vi "ex_readTdmChannelInfo.vi"(3 "error in (no error)":errorcluster, 4 "read info in":T4) -> (0 "error out":errorcluster, 1 "read info out":T4, 2 "comment":string)   [LabVIEW 2017]
uses:
  <vilib>/Platform/express/TDMExpress.llb/ex_readInfoTDM.ctl
  <vilib>/Platform/express/TDMExpress.llb/ex_readChannelInfo.ctl
  <vilib>/express/express shared/ExFile.llb/ex_TdmData.ctl
  <vilib>/express/express shared/ExFile.llb/ex_TdmProperty.ctl
  <vilib>/express/express shared/ex_EditUserDefinedProperties/usiDataType.ctl
  <vilib>/Platform/storage/lvStorage.llb/_wf_attributes.ctl
  <vilib>/Platform/storage/Storage.llb/__loadPropString.vi
  <vilib>/Platform/storage/Storage.llb/__loadPropRefList.vi
  <vilib>/Platform/storage/Storage.llb/__loadPropFloat64.vi
  <vilib>/Platform/storage/Storage.llb/__loadPropTime.vi
panel:
  out "Array":T1(array[cluster])
  in  "channel info":T2={"data chn ref"=refnum, "time chn ref"=refnum, "isRelativeTime ?"=FALSE, "channel length"=0, "dT"=0.0, "waveform stub"={"t0"=timestamp(0 s since 1904-01-01), "dt"=0.0, "Y"=[]}, "datatype"="", "timestamp"=timestamp(0 s since 1904-01-01)}
  in  "All Express Wave Attributes Plus PLUS":T3={"Start Timestamp"=timestamp(3198762007.7559996 s since 1904-01-01), "Timestamp"=timestamp(3198762007.8559995 s since 1904-01-01), "Relative Time?"=TRUE, "X Dimension"="f", "Signal Name"="Sawtooth with Uniform Noise (Power Spectrum)", "Y Units"="", "X0"=timestamp(0 s since 1904-01-01), "dX"=10.0, "nPoints"=50, "refnum"=refnum, "datatype"=""} {"dX" format="%.2f"; "X0" format="%<%X\n%x>T"; "Timestamp" format="%<%X\n%x>T"; "Start Timestamp" format="%<%X\n%x>T"}
  in  "Empty waveform":waveform(dbl)
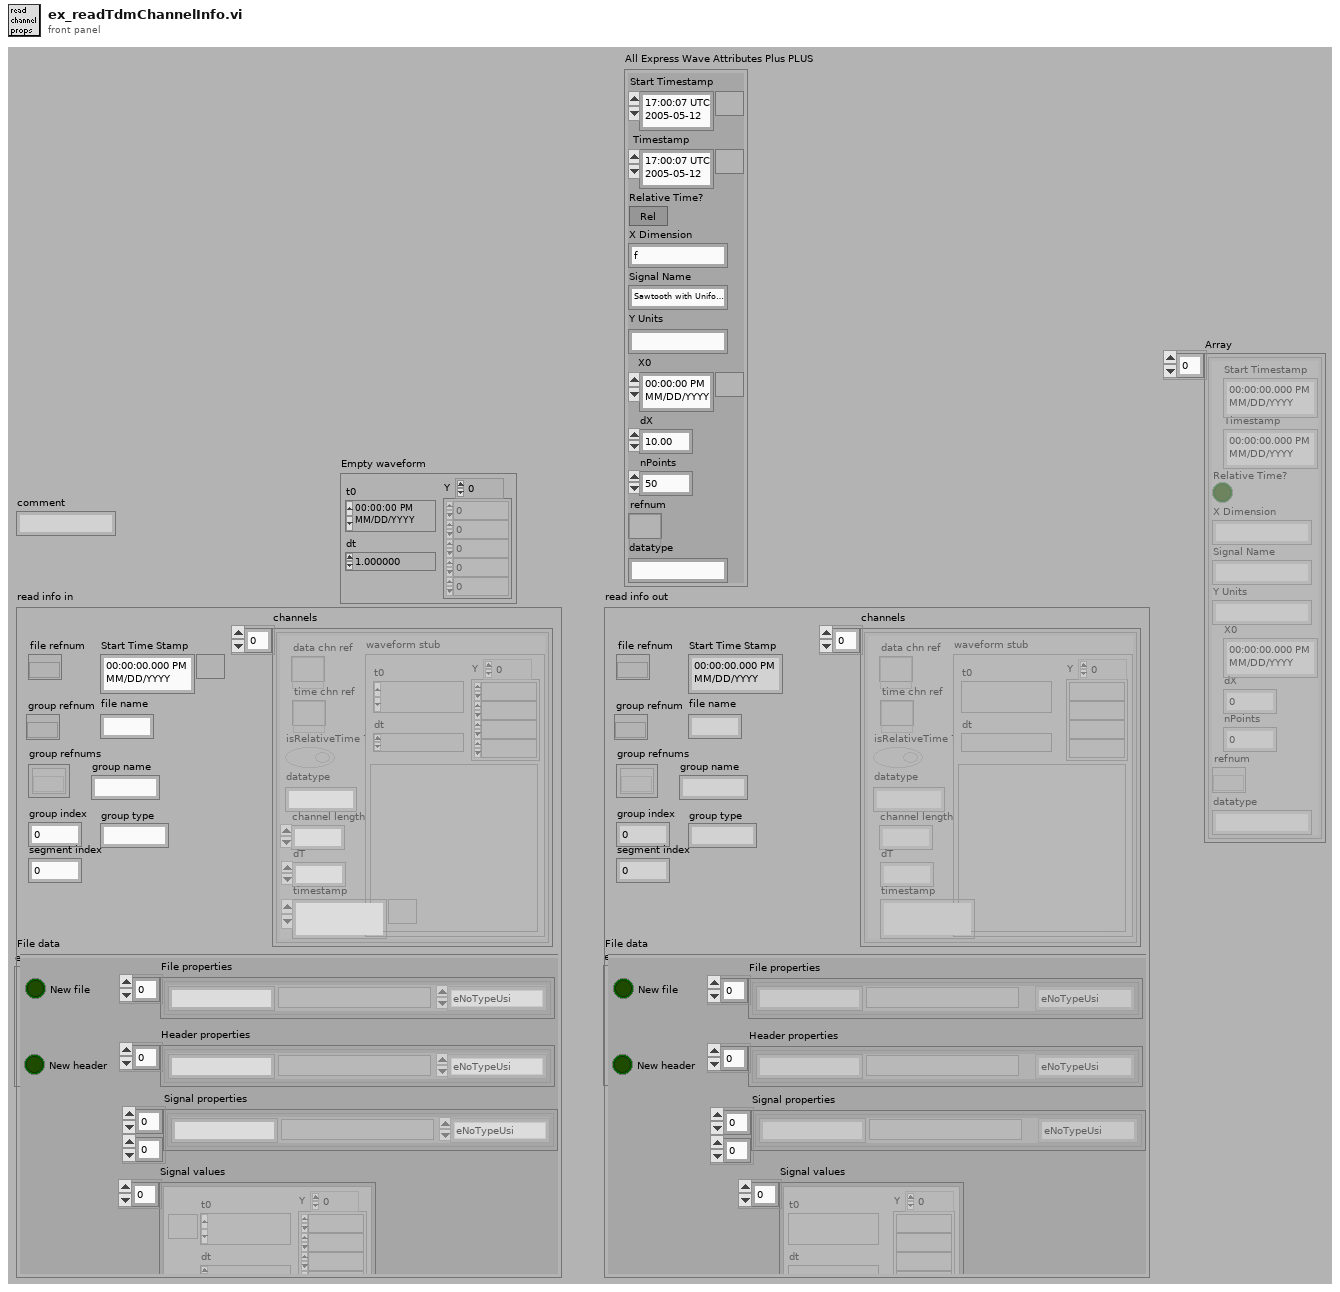
[diagram p1: front panel]
types:
  T1 = cluster{"Start Timestamp":timestamp, "Timestamp":timestamp, "Relative Time?":bool, "X Dimension":string, "Signal Name":string, "Y Units":string, "X0":timestamp, "dX":dbl, "nPoints":i32, "refnum":refnum<k20>, "datatype":string}[]
  T2 = typedef "ex_readChannelInfo.ctl" = cluster{"data chn ref":refnum<k20>, "time chn ref":refnum<k20>, "isRelativeTime ?":bool, "channel length":u32, "dT":dbl, "waveform stub":waveform(dbl), "datatype":string, "timestamp":timestamp}
  T3 = cluster{"Start Timestamp":timestamp, "Timestamp":timestamp, "Relative Time?":bool, "X Dimension":string, "Signal Name":string, "Y Units":string, "X0":timestamp, "dX":dbl, "nPoints":i32, "refnum":refnum<k20>, "datatype":string}
  T4 = typedef "ex_readInfoTDM.ctl" = cluster{"file refnum":refnum<k20>, "group refnum":refnum<k20>, "group name":string, "group type":string, "Start Time Stamp":timestamp, "group index":u32, "group refnums":refnum<k20>[], "file name":string, "segment index":u32, "channels":T2[], "File data":T5}
  T5 = typedef "ex_TdmData.ctl" = cluster{"New file":bool, "New header":bool, "File properties":T6[], "Header properties":T6[], "Signal properties":T6[][], "Signal values":waveform(dbl)[]}
  T6 = typedef "ex_TdmProperty.ctl" = cluster{"Name":string, "Type":T7, "Value":variant}
  T7 = typedef "usiDataType.ctl" = enum16{"eNoTypeUsi", "eInt8Usi", "eInt16Usi", "eInt32Usi", "eInt64Usi", "eUInt8Usi", "eUInt16Usi", "eUInt32Usi", "eUInt64Usi", "eFloat32Usi", "eFloat64Usi", "- 0", "- 1", "- 2", "- 3", "- 4", "- 5", "- 6", "- 7", "- 8", "- 9", "eString8Usi", "eString16Usi", "eStringUsi", "eEnumUsi", "- 10", "- 11", "- 12", "- 13", "- 14", "eTimeUsi", "- 15", "- 16", "- 17", "- 18", "- 19", "- 20", "- 21", "- 22", "- 23", "eInstanceUsi", "eStoreUsi"}
  T8 = typedef "_wf_attributes.ctl" = enum16{"t0", "dt", "X_Name", "X_Unit", "x0", "abs/rel", "nPoints", "file_timestamp", "xcolumns"}
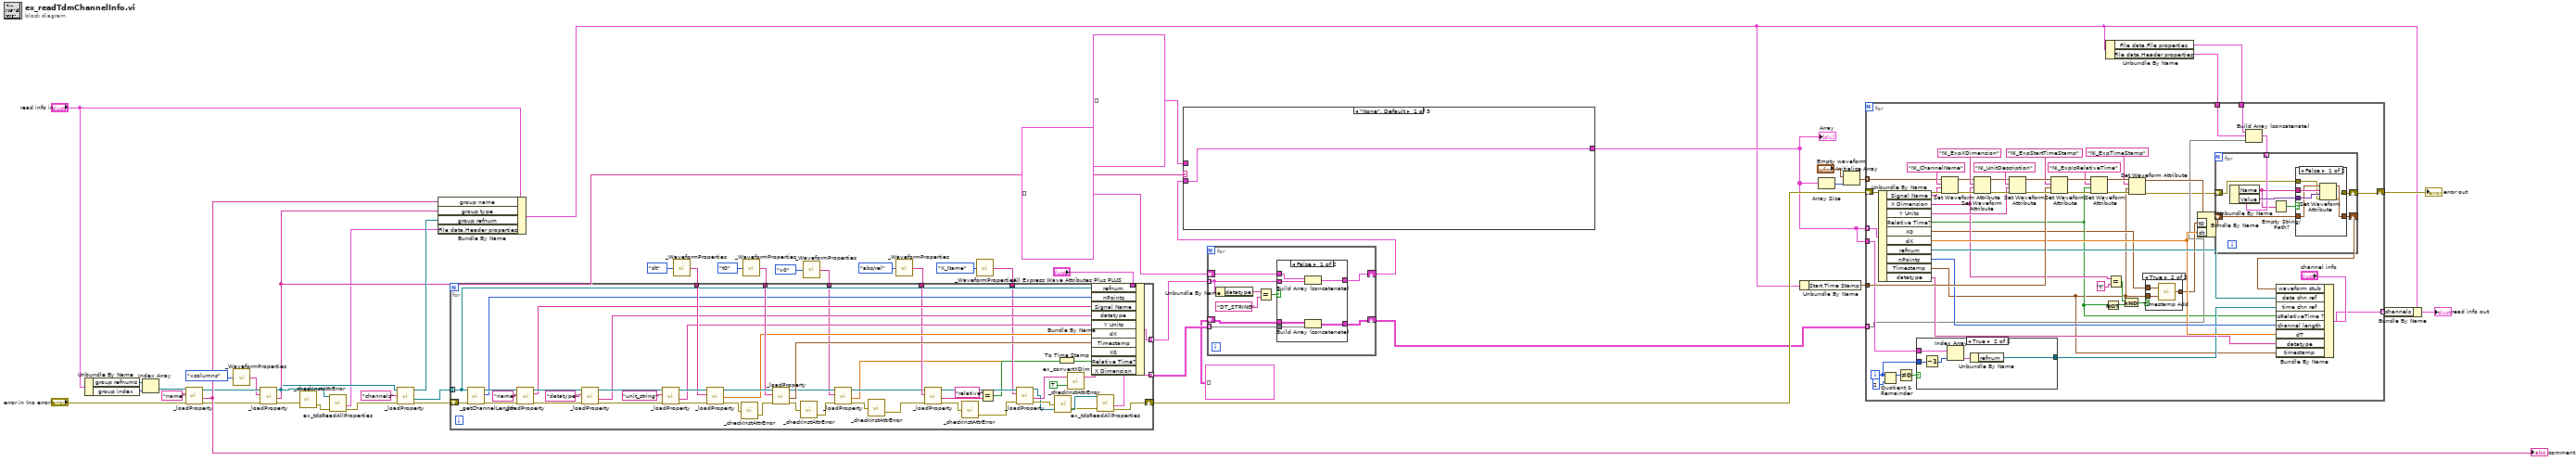
[diagram p0: block diagram]
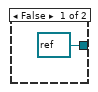
[diagram p5: hidden frame]
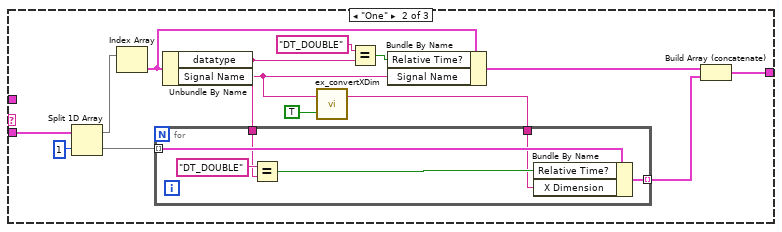
[diagram p6: hidden frame]
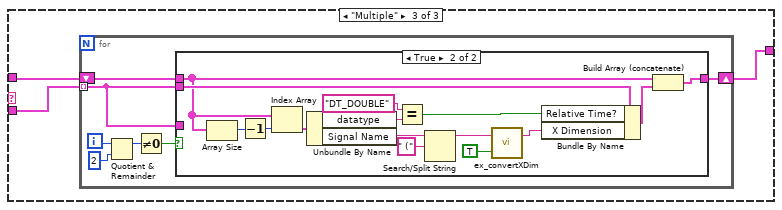
[diagram p7: hidden frame]
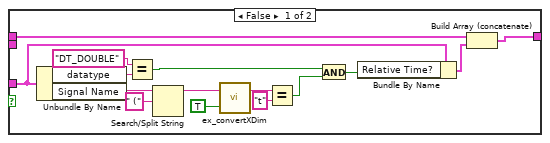
[diagram p8: hidden frame]
diagram:
  n1 = Unbundle By Name("read info in") -> ("group refnums"=w41:refnum<k20>[], "group index"=w50:u32)
  n2 = Index Array(array=w41, index=w50) -> (element=w42:refnum<k20>)
  n3 = call-poly <vilib>:"_loadProperty.vi"("error in (no error)"="error in (no error)", "Property name"="name", "storage refnum"=w42) -> ("error out"=w45:errorcluster, "Value"=w51:string, "dup storage refnum"=w46:refnum<k20>)  [unwired: 6 out]
  "comment" <- w51
  n4 = call <vilib>:"_WaveformProperties.vi"("Property"=_wf_attributes."xcolumns") -> ("Name"=w43:string)
  n5 = call-poly <vilib>:"_loadProperty.vi"("error in (no error)"=w45, "Property name"=w43, "storage refnum"=w46) -> ("error out"=w18:errorcluster, "Value"=w36:string, "dup storage refnum"=w14:refnum<k20>)  [unwired: 6 out]
  n6 = call <vilib>:"_checkInstAttrError.vi"("error in (no error)"=w18) -> ("error out"=w13:errorcluster)  [unwired: 1 out]
  n7 = call <vilib>:"ex_tdsReadAllProperties.vi"("error in (no error)"=w13, "Data Object in"=w14) -> ("error out"=w12:errorcluster, "Properties Out"=w11:T6[])  [unwired: 4 out]
  n8 = call-poly <vilib>:"_loadProperty.vi"("error in (no error)"=w12, "Property name"="channels", "storage refnum"=w14) -> ("error out"=w39:errorcluster, "Value"=w40:refnum<k20>[], "dup storage refnum"=w38:refnum<k20>)  [unwired: 6 out]
  n9 = Bundle By Name(cluster="read info in", "group name"=w51, "group type"=w36, "group refnum"=w38, "File data.Header properties"=w11) -> (w9:T4)
  n10 = call <vilib>:"_WaveformProperties.vi"("Property"=_wf_attributes."dt") -> ("Name"=w27:string)
  n11 = call <vilib>:"_WaveformProperties.vi"("Property"=_wf_attributes."t0") -> ("Name"=w25:string)
  n12 = call <vilib>:"_WaveformProperties.vi"("Property"=_wf_attributes."x0") -> ("Name"=w15:string)
  n13 = call <vilib>:"_WaveformProperties.vi"("Property"=_wf_attributes."abs/rel") -> ("Name"=w22:string)
  n14 = call <vilib>:"_WaveformProperties.vi"("Property"=_wf_attributes."X_Name") -> ("Name"=w19:string)
  n15 = for {
    shift-right: [w53] -> w32
    shift-left: w39 -> [w102]
    tunnel: w40 -> [w76] mode=indexing
    tunnel: w27 -> [w91]
    tunnel: w25 -> [w89]
    tunnel: "All Express Wave Attributes Plus PLUS" -> [w87]
    tunnel: w22 -> [w80]
    tunnel: [w77] -> w5 mode=indexing
    tunnel: w19 -> [w74]
    tunnel: w15 -> [w59]
    tunnel: [w52] -> w3 mode=indexing
    n16 = call <vilib>:"_getChannelLength.vi"("error in (no error)"=w102, "channel refnum in"=w76) -> ("error out"=w99:errorcluster, "channel length"=w86:i32, "channel refnum out"=w98:refnum<k20>)  [unwired: 3 out]
    n17 = call-poly <vilib>:"_loadProperty.vi"("error in (no error)"=w99, "Property name"="name", "storage refnum"=w98) -> ("error out"=w97:errorcluster, "Value"=w85:string, "dup storage refnum"=w96:refnum<k20>)  [unwired: 1 in, 5 out]
    n18 = call-poly <vilib>:"_loadProperty.vi"("error in (no error)"=w97, "Property name"="datatype", "storage refnum"=w96) -> ("error out"=w94:errorcluster, "Value"=w84:string, "dup storage refnum"=w93:refnum<k20>)  [unwired: 1 in, 5 out]
    n19 = call-poly <vilib>:"_loadProperty.vi"("error in (no error)"=w94, "Property name"="unit_string", "storage refnum"=w93) -> ("error out"=w88:errorcluster, "Value"=w83:string, "dup storage refnum"=w92:refnum<k20>)  [unwired: 1 in, 5 out]
    n20 = call-poly <vilib>:"_loadProperty.vi"("error in (no error)"=w88, "Property name"=w91, "storage refnum"=w92) -> ("error out"=w70:errorcluster, "Value"=w82:dbl, "dup storage refnum"=w90:refnum<k20>)  [unwired: 6 out]
    n21 = call <vilib>:"_checkInstAttrError.vi"("error in (no error)"=w70) -> ("error out"=w69:errorcluster)  [unwired: 1 out]
    n22 = call-poly <vilib>:"_loadProperty.vi"("error in (no error)"=w69, "Property name"=w89, "storage refnum"=w90) -> ("error out"=w68:errorcluster, "Value"=w81:timestamp, "dup storage refnum"=w61:refnum<k20>)  [unwired: 6 out]
    n23 = call <vilib>:"_checkInstAttrError.vi"("error in (no error)"=w68) -> ("error out"=w63:errorcluster)  [unwired: 1 out]
    n24 = call-poly <vilib>:"_loadProperty.vi"("error in (no error)"=w63, "Property name"=w59, "storage refnum"=w61) -> ("error out"=w64:errorcluster, "Value"=w56:dbl, "dup storage refnum"=w60:refnum<k20>)  [unwired: 6 out]
    n25 = call <vilib>:"_checkInstAttrError.vi"("error in (no error)"=w64) -> ("error out"=w62:errorcluster)  [unwired: 1 out]
    n26 = call-poly <vilib>:"_loadProperty.vi"("error in (no error)"=w62, "Property name"=w80, "storage refnum"=w60) -> ("error out"=w67:errorcluster, "Value"=w79:string, "dup storage refnum"=w75:refnum<k20>)  [unwired: 6 out]
    n27 = call <vilib>:"_checkInstAttrError.vi"("error in (no error)"=w67) -> ("error out"=w66:errorcluster)  [unwired: 1 out]
    n28 = Equal?(x="relative", y=w79) -> (x = y?=w58:bool)
    n29 = call-poly <vilib>:"_loadProperty.vi"("error in (no error)"=w66, "Property name"=w74, "storage refnum"=w75) -> ("error out"=w65:errorcluster, "Value"=w72:string, "dup storage refnum"=w55:refnum<k20>)  [unwired: 6 out]
    n30 = call <vilib>:"_checkInstAttrError.vi"("error in (no error)"=w65) -> ("error out"=w54:errorcluster)  [unwired: 1 out]
    n31 = To Time Stamp(1:w56) -> (0:w57:timestamp)
    n32 = call <vilib>:"ex_convertXDim.vi"("mode (F:Code to String)"=TRUE, "x_dimension in"=w72) -> ("x_dimension out"=w71:string)  [unwired: 1 out]
    n33 = Bundle By Name(cluster=w87, "refnum"=w76, "nPoints"=w86, "Signal Name"=w85, "datatype"=w84, "Y Units"=w83, "dX"=w82, "Timestamp"=w81, "X0"=w57, "Relative Time?"=w58, "X Dimension"=w71) -> (w77:T3)
    n34 = call <vilib>:"ex_tdsReadAllProperties.vi"("error in (no error)"=w54, "Data Object in"=w55) -> ("error out"=w53:errorcluster, "Properties Out"=w52:T6[])  [unwired: 4 out]
  }
  n35 = for {
    tunnel: w5 -> [w108] mode=indexing
    shift-right: [w107] -> w4
    shift-left: T1 [] ("Array 2") -> [w106]
    tunnel: w3 -> [w105] mode=indexing
    shift-right: [w104] -> w1
    shift-left: T6[][] [] ("Properties Out") -> [w103]
    n36 = Unbundle By Name(w108) -> ("datatype"=w111:string)
    n37 = Equal?(x=w111, y="DT_STRING") -> (x = y?=w109:bool)
    n38 = case shown="False" w109 {
      tunnel: w108 -> [w117 _]
      tunnel: [w116 w119] -> w107
      tunnel: w106 -> [w115 w119]
      tunnel: w105 -> [w114 _]
      tunnel: [w113 w118] -> w104
      tunnel: w103 -> [w112 w118]
      frame False {
        n39 = Build Array (concatenate)(w115, w117) -> (w116:T1)
        n40 = Build Array (concatenate)(w112, w114) -> (w113:T6[][])
      }
      frame True {
      }
    }
  }
  n41 = case shown="\"None\", Default" w36 {
    tunnel: w4 -> [w120 w132 w142]
    tunnel: [w120 w123 w141] -> w10
    tunnel: T1 [] -> [_ _ w143]
    frame "None", Default {
    }
    frame "One" {
      n42 = Split 1D Array(array=w132, index=1) -> (first subarray=w131:T1, second subarray=w129:T1)
      n43 = Index Array(array=w131) -> (element=w130:T3)  [unwired: 1 in]
      n44 = Unbundle By Name(w130) -> ("datatype"=w127:string, "Signal Name"=w121:string)
      n45 = call <vilib>:"ex_convertXDim.vi"("mode (F:Code to String)"=TRUE, "x_dimension in"=w121) -> ("x_dimension out"=w125:string)  [unwired: 1 out]
      n46 = for {
        tunnel: w129 -> [w140] mode=indexing
        tunnel: [w138] -> w124 mode=indexing
        tunnel: w127 -> [w136]
        tunnel: w125 -> [w135]
        n47 = Equal?(x="DT_DOUBLE", y=w136) -> (x = y?=w139:bool)
        n48 = Bundle By Name(cluster=w140, "Relative Time?"=w139, "X Dimension"=w135) -> (w138:T3)
      }
      n49 = Equal?(x="DT_DOUBLE", y=w127) -> (x = y?=w126:bool)
      n50 = Bundle By Name(cluster=w130, "Relative Time?"=w126, "Signal Name"=w121) -> (w122:T3)
      n51 = Build Array (concatenate)(w122, w124) -> (w123:T1)
    }
    frame "Multiple" {
      n52 = for {
        shift-right: [w147] -> w141
        shift-left: w143 -> [w148]
        tunnel: w142 -> [w145] mode=indexing
        i -> [w144]
        n53 = Quotient & Remainder(x=w144, y=2) -> (x-y*floor(x/y)=w146:i32)  [unwired: 1 out]
        n54 = Not Equal To 0?(x=w146) -> (x != 0?=w149:bool)
        n55 = case shown="True" w149 {
          tunnel: w148 -> [w157 w171]
          tunnel: [w156 w180] -> w147
          tunnel: w145 -> [_ w177]
          tunnel: w145 -> [w158 _]
          frame False {
            n56 = Unbundle By Name(w158) -> ("datatype"=w164:string, "Signal Name"=w160:string)
            n57 = Equal?(x="DT_DOUBLE", y=w164) -> (x = y?=w155:bool)
            n58 = Search/Split String(string=w160, search string/char (-)=" (") -> (substring before match=w163:string)  [unwired: 3 out]
            n59 = call <vilib>:"ex_convertXDim.vi"("mode (F:Code to String)"=TRUE, "x_dimension in"=w163) -> ("x_dimension out"=w153:string)  [unwired: 1 out]
            n60 = Equal?(x=w153, y="t") -> (x = y?=w152:bool)
            n61 = And(x=w155, y=w152) -> (x .and. y?=w154:bool)
            n62 = Bundle By Name(cluster=w158, "Relative Time?"=w154) -> (w159:T3)
            n63 = Build Array (concatenate)(w157, w159) -> (w156:T1)
          }
          frame True {
            n64 = Array Size(array=w171) -> (size(s)=w172:i32)
            n65 = Decrement(x=w172) -> (x-1=w175:i32)
            n66 = Index Array(array=w171, index=w175) -> (element=w174:T3)
            n67 = Unbundle By Name(w174) -> ("datatype"=w173:string, "Signal Name"=w167:string)
            n68 = Equal?(x="DT_DOUBLE", y=w173) -> (x = y?=w178:bool)
            n69 = Search/Split String(string=w167, search string/char (-)=" (") -> (substring before match=w170:string)  [unwired: 3 out]
            n70 = call <vilib>:"ex_convertXDim.vi"("mode (F:Code to String)"=TRUE, "x_dimension in"=w170) -> ("x_dimension out"=w166:string)  [unwired: 1 out]
            n71 = Bundle By Name(cluster=w177, "Relative Time?"=w178, "X Dimension"=w166) -> (w176:T3)
            n72 = Build Array (concatenate)(w171, w176) -> (w180:T1)
          }
        }
      }
    }
  }
  "Array" <- w10
  n73 = Unbundle By Name(w9) -> ("Start Time Stamp"=w30:timestamp)
  n74 = Array Size(array=w10) -> (size(s)=w35:i32)
  n75 = Initialize Array("Empty waveform", w35) -> (w33:waveform(dbl)[])
  n76 = Unbundle By Name(w9) -> ("File data.File properties"=w8:T6[], "File data.Header properties"=w7:T6[])
  n77 = for {
    tunnel: w33 -> [w219] mode=indexing
    shift-right: [w181] -> w31
    shift-left: w32 -> [w218]
    tunnel: w30 -> [w217]
    tunnel: w10 -> [w202] mode=indexing
    tunnel: [w206] -> w17 mode=indexing
    tunnel: w10 -> [w201]
    tunnel: w1 -> [w185] mode=indexing
    tunnel: w8 -> [w187]
    tunnel: w7 -> [w186]
    i -> [w200]
    n78 = Unbundle By Name(w202) -> ("Signal Name"=w216:string, "X Dimension"=w195:string, "Y Units"=w215:string, "Relative Time?"=w193:bool, "X0"=w192:timestamp, "dX"=w207:dbl, "refnum"=w209:refnum<k20>, "nPoints"=w208:i32, "Timestamp"=w189:timestamp, "datatype"=w190:string)
    n79 = Quotient & Remainder(x=w200, y=2) -> (x-y*floor(x/y)=w205:i32)  [unwired: 1 out]
    n80 = Not Equal To 0?(x=w205) -> (x != 0?=w203:bool)
    n81 = case shown="True" w203 {
      tunnel: w201 -> [_ w258]
      tunnel: w200 -> [_ w256]
      tunnel: [refnum<k20> refnum ("refnum") w254] -> w199
      frame False {
      }
      frame True {
        n82 = Decrement(x=w256) -> (x-1=w257:i32)
        n83 = Index Array(array=w258, index=w257) -> (element=w255:T3)
        n84 = Unbundle By Name(w255) -> ("refnum"=w254:refnum<k20>)
      }
    }
    n85 = Set Waveform Attribute(4:w218, 5:w216, 6:"NI_ChannelName" ("name"), 7:w219) -> (0:w222:errorcluster, 3:w223:waveform(dbl))  [unwired: 1 out]
    n86 = Set Waveform Attribute(4:w222, 5:w195, 6:"NI_ExpXDimension" ("name"), 7:w223) -> (0:w220:errorcluster, 3:w221:waveform(dbl))  [unwired: 1 out]
    n87 = Set Waveform Attribute(4:w220, 5:w215, 6:"NI_UnitDescription" ("name"), 7:w221) -> (0:w228:errorcluster, 3:w229:waveform(dbl))  [unwired: 1 out]
    n88 = Set Waveform Attribute(4:w228, 5:w217, 6:"NI_ExpStartTimeStamp" ("name"), 7:w229) -> (0:w231:errorcluster, 3:w232:waveform(dbl))  [unwired: 1 out]
    n89 = Set Waveform Attribute(4:w231, 5:w193, 6:"NI_ExpIsRelativeTime" ("name"), 7:w232) -> (0:w214:errorcluster, 3:w213:waveform(dbl))  [unwired: 1 out]
    n90 = Not(x=w193) -> (.not. x?=w196:bool)
    n91 = Equal?(x=w195, y="t") -> (x = y?=w191:bool)
    n92 = And(x=w191, y=w196) -> (x .and. y?=w197:bool)
    n93 = Set Waveform Attribute(4:w214, 5:w189, 6:"NI_ExpTimeStamp" ("name"), 7:w213) -> (0:w182:errorcluster, 3:w212:waveform(dbl))  [unwired: 1 out]
    n94 = case shown="True" w197 {
      tunnel: w192 -> [w249 w252]
      tunnel: w189 -> [_ w251]
      tunnel: [w249 w250] -> w194
      frame False {
      }
      frame True {
        n95 = call <vilib>:"Timestamp Add.vi"("y"=w251, "x"=w252) -> ("x + y"=w250:timestamp)
      }
    }
    n96 = Bundle By Name(cluster=w212, "t0"=w194, "dt"=w207) -> (w183:waveform(dbl))
    n97 = Build Array (concatenate)(w187, w186, w185) -> (w184:T6[])
    n98 = for {
      tunnel: w184 -> [w238] mode=indexing
      shift-right: [w240] -> w188
      shift-left: w183 -> [w237]
      shift-right: [w233] -> w181
      shift-left: w182 -> [w234]
      n99 = Unbundle By Name(w238) -> ("Name"=w236:string, "Value"=w239:variant)
      n100 = Empty String/Path?(string/path=w236) -> (empty?=w235:bool)
      n101 = case shown="False" w235 {
        tunnel: [w246 w248] -> w240
        tunnel: w239 -> [w245 _]
        tunnel: w236 -> [w244 _]
        tunnel: w237 -> [w243 w248]
        tunnel: w234 -> [w242 w247]
        tunnel: [w241 w247] -> w233
        frame False {
          n102 = Set Waveform Attribute(4:w242, 5:w245, 6:w244, 7:w243) -> (0:w241:errorcluster, 3:w246:waveform(dbl))  [unwired: 1 out]
        }
        frame True {
        }
      }
    }
    n103 = Bundle By Name(cluster="channel info", "waveform stub"=w188, "data chn ref"=w209, "time chn ref"=w199, "isRelativeTime ?"=w193, "channel length"=w208, "dT"=w207, "datatype"=w190, "timestamp"=w189) -> (w206:T2)
  }
  "error out" <- w31
  n104 = Bundle By Name(cluster=w9, "channels"=w17) -> (→"read info out":T4)
